vi "cam2 analyse.vi"() -> (0 "W6 chiffre":string, 1 "O6 chiffre":string, 2 "G1 chiffre":string, 3 "G4 chiffre":string, 4 "G8 chiffre":string, 5 "W9 chiffre":string, 7 "W8 chiffre":string, 9 "W7 chiffre":string, 11 "O3 chiffre":string, 12 "O9 chiffre":string, 13 "G2 chiffre":string, 14 "G7 chiffre":string)   [LabVIEW 2019]
uses:
  <vilib>/vision/Classification.llb/IMAQ Classifier Read Options.ctl
  <vilib>/vision/NI_Vision_Development_Module.lvlib
panel:
  in  "error in":errorcluster
  out "Coordinates":i32[](array[numeric])
  in  "G8":T1={"Global Rectangle"=[0, 0, 1279, 959], "Contours"=[{"ID"=enum."External", "Type"=3, "Coordinates"=[0, 0, 1279, 959]}]} {"Contours"."Type" items=["No Selection", "Point", "Line", "Rectangle", "Oval", "Polygon", "Freehand Region", "Annulus", "Unused2", "Unused3", "Broken Line", "Freehand Line", "Rotated Rectangle"]}
  out "G8":string[](array[string])
  in  "G7":T1={"Global Rectangle"=[0, 0, 1279, 959], "Contours"=[{"ID"=enum."External", "Type"=3, "Coordinates"=[0, 0, 1279, 959]}]} {"Contours"."Type" items=["No Selection", "Point", "Line", "Rectangle", "Oval", "Polygon", "Freehand Region", "Annulus", "Unused2", "Unused3", "Broken Line", "Freehand Line", "Rotated Rectangle"]}
  out "G7":string[](array[string])
  in  "G4":T1={"Global Rectangle"=[0, 0, 1279, 959], "Contours"=[{"ID"=enum."External", "Type"=3, "Coordinates"=[0, 0, 1279, 959]}]} {"Contours"."Type" items=["No Selection", "Point", "Line", "Rectangle", "Oval", "Polygon", "Freehand Region", "Annulus", "Unused2", "Unused3", "Broken Line", "Freehand Line", "Rotated Rectangle"]}
  out "G4":string[](array[string])
  in  "G2":T1={"Global Rectangle"=[0, 0, 1279, 959], "Contours"=[{"ID"=enum."External", "Type"=3, "Coordinates"=[0, 0, 1279, 959]}]} {"Contours"."Type" items=["No Selection", "Point", "Line", "Rectangle", "Oval", "Polygon", "Freehand Region", "Annulus", "Unused2", "Unused3", "Broken Line", "Freehand Line", "Rotated Rectangle"]}
  out "G2":string[](array[string])
  in  "G1":T1={"Global Rectangle"=[0, 0, 1279, 959], "Contours"=[{"ID"=enum."External", "Type"=3, "Coordinates"=[0, 0, 1279, 959]}]} {"Contours"."Type" items=["No Selection", "Point", "Line", "Rectangle", "Oval", "Polygon", "Freehand Region", "Annulus", "Unused2", "Unused3", "Broken Line", "Freehand Line", "Rotated Rectangle"]}
  out "G1":string[](array[string])
  in  "O9":T1={"Global Rectangle"=[0, 0, 1279, 959], "Contours"=[{"ID"=enum."External", "Type"=3, "Coordinates"=[0, 0, 1279, 959]}]} {"Contours"."Type" items=["No Selection", "Point", "Line", "Rectangle", "Oval", "Polygon", "Freehand Region", "Annulus", "Unused2", "Unused3", "Broken Line", "Freehand Line", "Rotated Rectangle"]}
  out "O9":string[](array[string])
  in  "O6":T1={"Global Rectangle"=[0, 0, 1279, 959], "Contours"=[{"ID"=enum."External", "Type"=3, "Coordinates"=[0, 0, 1279, 959]}]} {"Contours"."Type" items=["No Selection", "Point", "Line", "Rectangle", "Oval", "Polygon", "Freehand Region", "Annulus", "Unused2", "Unused3", "Broken Line", "Freehand Line", "Rotated Rectangle"]}
  out "O6":string[](array[string])
  in  "O3":T1={"Global Rectangle"=[0, 0, 1279, 959], "Contours"=[{"ID"=enum."External", "Type"=3, "Coordinates"=[0, 0, 1279, 959]}]} {"Contours"."Type" items=["No Selection", "Point", "Line", "Rectangle", "Oval", "Polygon", "Freehand Region", "Annulus", "Unused2", "Unused3", "Broken Line", "Freehand Line", "Rotated Rectangle"]}
  out "O3":string[](array[string])
  in  "W7":T1={"Global Rectangle"=[0, 0, 1279, 959], "Contours"=[{"ID"=enum."External", "Type"=3, "Coordinates"=[0, 0, 1279, 959]}]} {"Contours"."Type" items=["No Selection", "Point", "Line", "Rectangle", "Oval", "Polygon", "Freehand Region", "Annulus", "Unused2", "Unused3", "Broken Line", "Freehand Line", "Rotated Rectangle"]}
  out "W7":string[](array[string])
  in  "W8":T1={"Global Rectangle"=[0, 0, 1279, 959], "Contours"=[{"ID"=enum."External", "Type"=3, "Coordinates"=[0, 0, 1279, 959]}]} {"Contours"."Type" items=["No Selection", "Point", "Line", "Rectangle", "Oval", "Polygon", "Freehand Region", "Annulus", "Unused2", "Unused3", "Broken Line", "Freehand Line", "Rotated Rectangle"]}
  out "W8":string[](array[string])
  in  "W9":T1={"Global Rectangle"=[0, 0, 1279, 959], "Contours"=[{"ID"=enum."External", "Type"=3, "Coordinates"=[0, 0, 1279, 959]}]} {"Contours"."Type" items=["No Selection", "Point", "Line", "Rectangle", "Oval", "Polygon", "Freehand Region", "Annulus", "Unused2", "Unused3", "Broken Line", "Freehand Line", "Rotated Rectangle"]}
  out "W9":string[](array[string])
  in  "W6":T1={"Global Rectangle"=[640, 450, 686, 504], "Contours"=[{"ID"=enum."External", "Type"=3, "Coordinates"=[640, 450, 686, 504]}]} {"Contours"."Type" items=["No Selection", "Point", "Line", "Rectangle", "Oval", "Polygon", "Freehand Region", "Annulus", "Unused2", "Unused3", "Broken Line", "Freehand Line", "Rotated Rectangle"]}
  out "Image Out 2":T2(plugin-control)
  out "W6":string[](array[string])
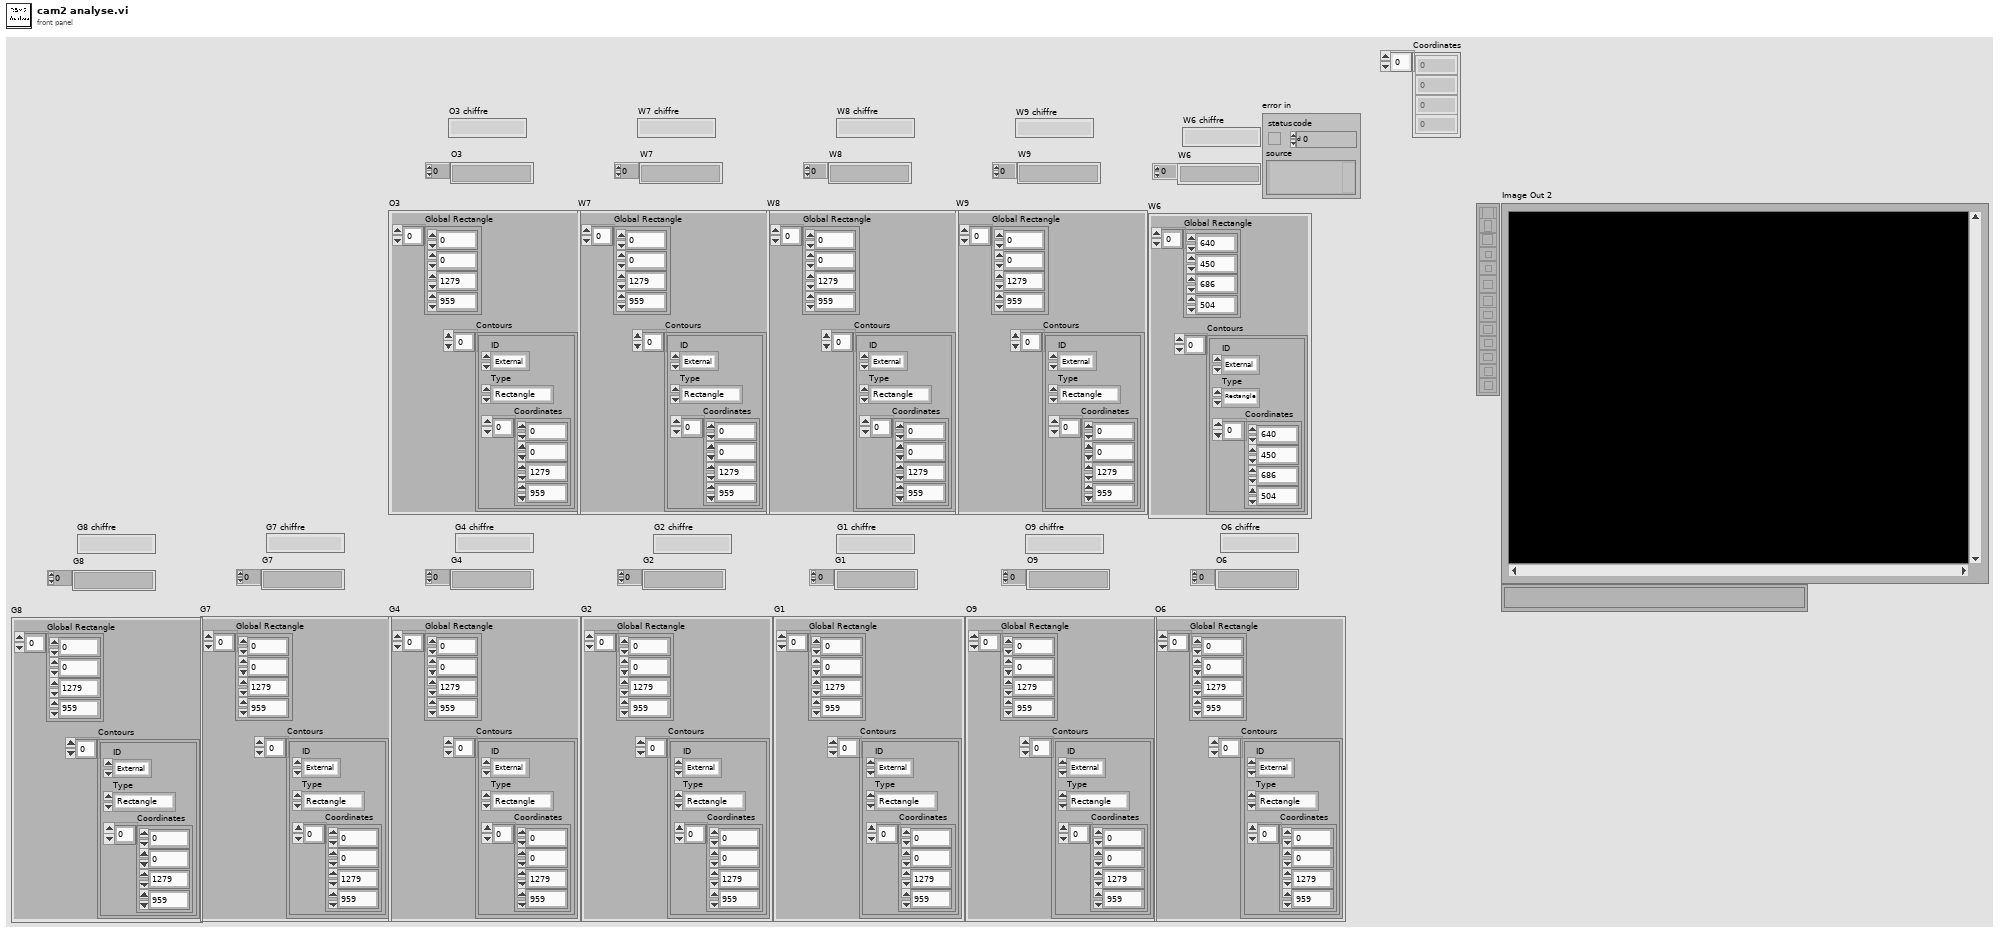
[diagram p1: front panel]
types:
  T1 = cluster{"Global Rectangle":i32[], "Contours":cluster{"ID":enum32{"External", "Internal"}, "Type":u32, "Coordinates":i32[]}[]}
  T2 = typedef "IMAQ Image.ctl" = refnum<image>
  T3 = typedef "IMAQ Classifier Read Options.ctl" = i32
  T4 = typedef "IMAQ Classifier Session.ctl" = refnum<k1>
  T5 = typedef "ROI Descriptor" = cluster{"Global Rectangle":i32[], "Contours":cluster{"ID":enum32{"External", "Internal"}, "Type":u32, "Coordinates":i32[]}[]}
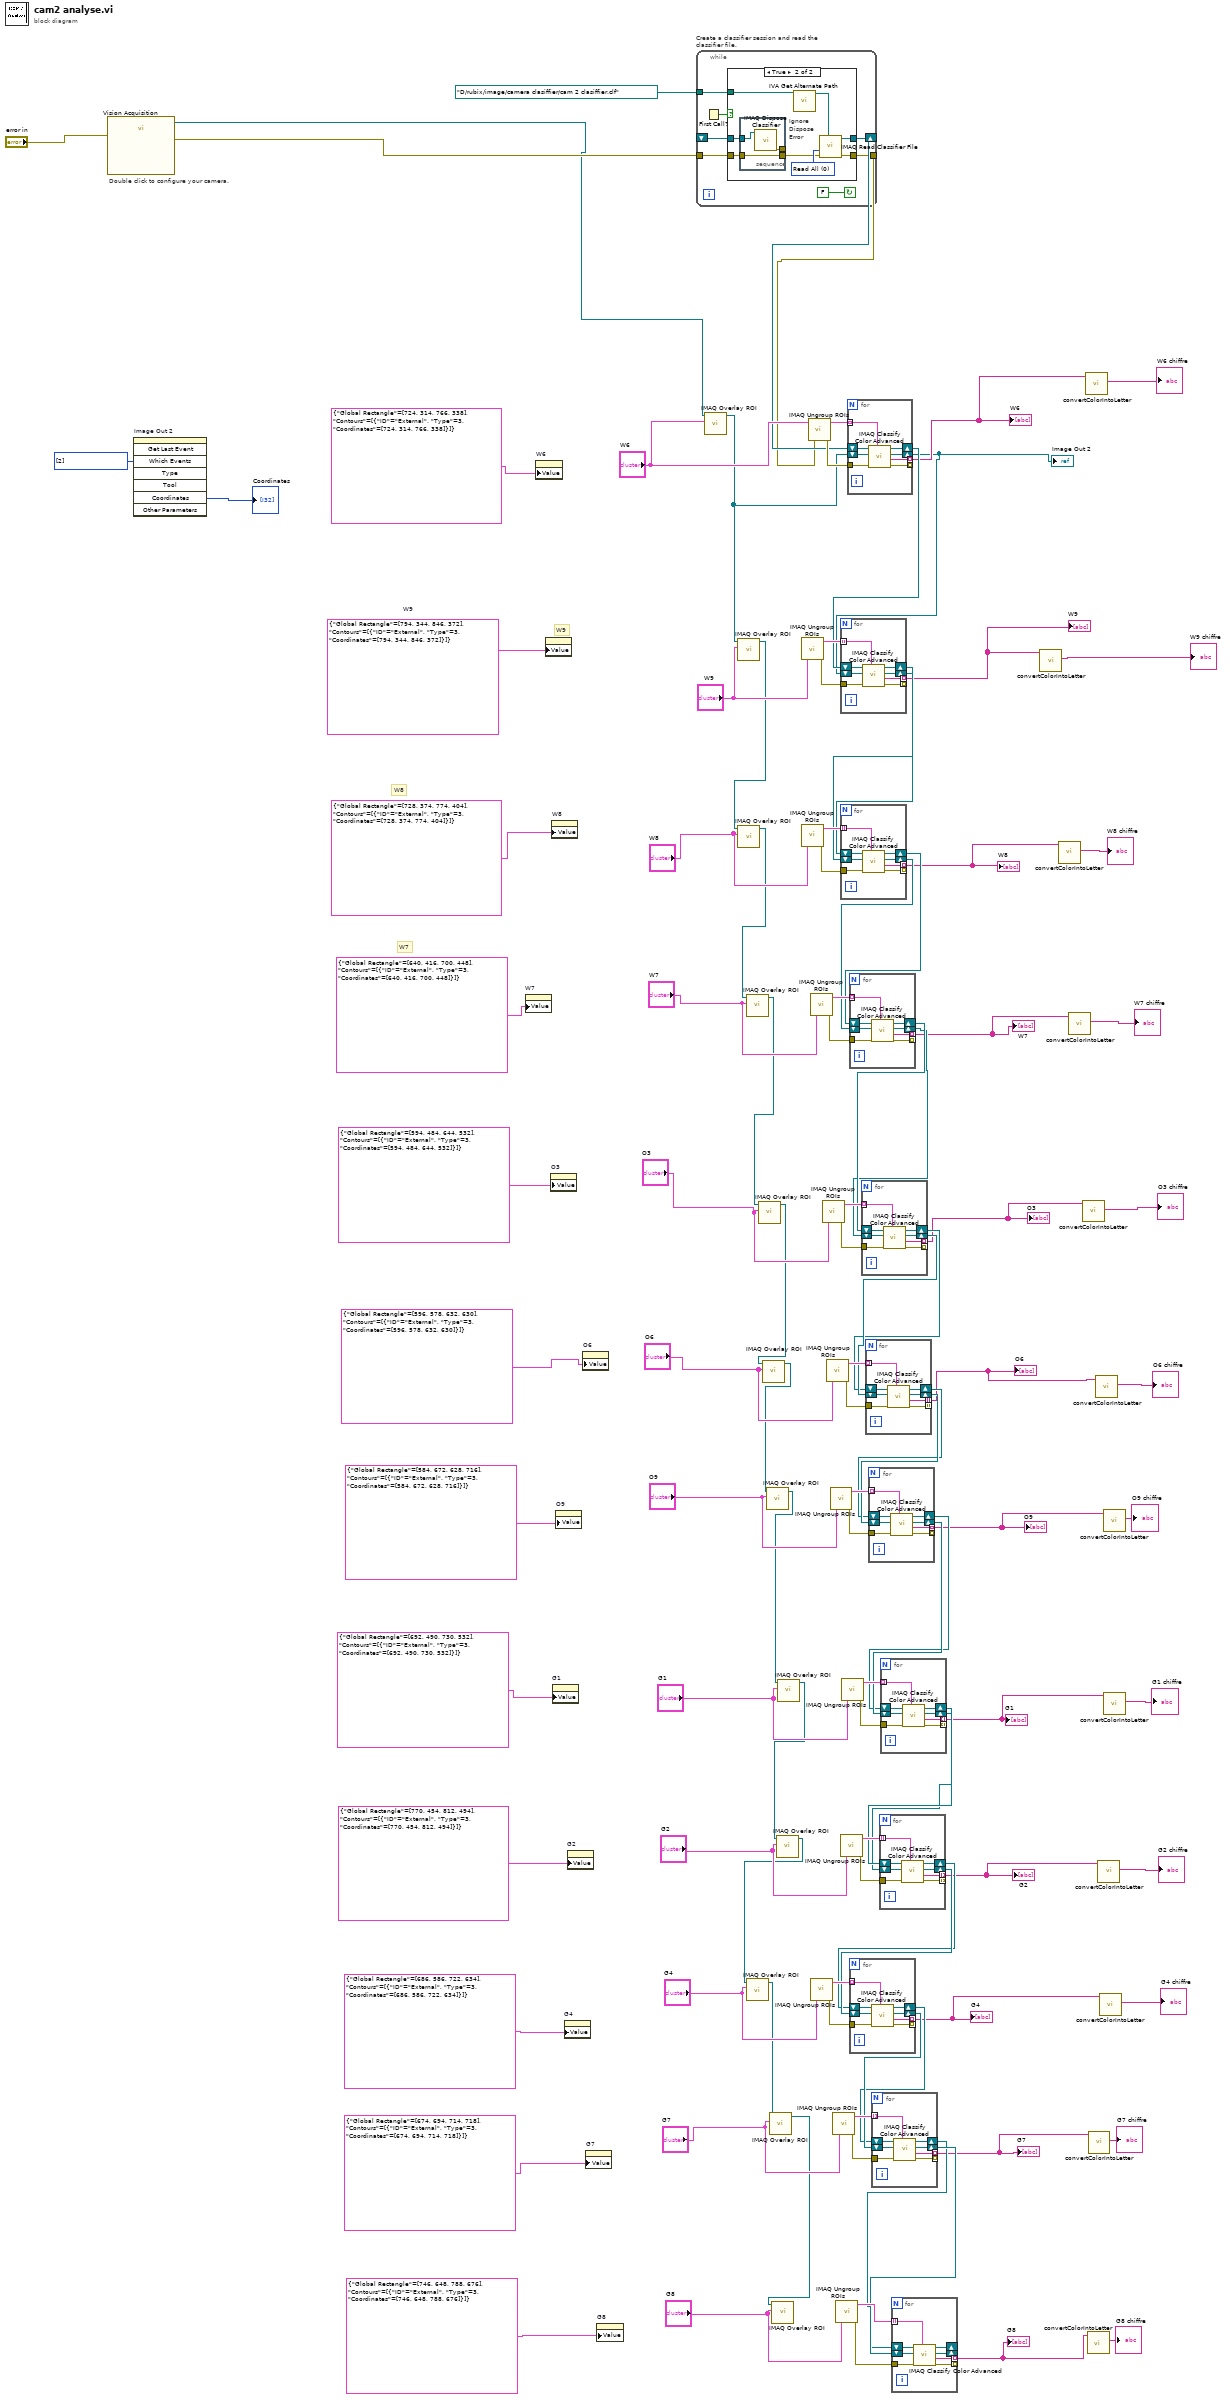
[diagram p0: block diagram]
diagram:
  w7 = i32[] [2] items=["No Event"=0, "Click Event"=1, "Draw Event"=2, "Size Event"=4, "Scroll Event"=5, "Double Click Event"=8] ("Which Events")
  # "W9"
  # "W7"
  # "W8"
  # "Double click to configure your camera."
  n1 = call "Vision Acquisition"("error in"="error in") -> ("Image Out"=w3:T2, "error out"=w113:errorcluster)  [unwired: 25 in]
  n2 = invoke on="Image Out 2" class="ImageControl" method="Get Last Event"("Which Events"=w7) -> ("Coordinates"=→"Coordinates":i32[])  [unwired: 7 in, 7 out]
  n3 = property on="W7" class="Clust (strict)"("Value"=T1 {"Global Rectangle"=[640, 416, 700, 448], "Contours"=[{"ID"=enum."External", "Type"=3, "Coordinates"=[640, 416, 700, 448]}]} ("ROI Descriptor (Color Classification 1)")) -> ()  [unwired: 2 in, 2 out]
  n4 = property on="W6" class="Clust (strict)"("Value"=T1 {"Global Rectangle"=[724, 314, 766, 338], "Contours"=[{"ID"=enum."External", "Type"=3, "Coordinates"=[724, 314, 766, 338]}]} ("ROI Descriptor (Color Classification 1)")) -> ()  [unwired: 2 in, 2 out]
  n5 = property on="W9" class="Clust (strict)"("Value"=T1 {"Global Rectangle"=[794, 344, 846, 372], "Contours"=[{"ID"=enum."External", "Type"=3, "Coordinates"=[794, 344, 846, 372]}]} ("ROI Descriptor (Color Classification 1)")) -> ()  [unwired: 2 in, 2 out]
  n6 = property on="O3" class="Clust (strict)"("Value"=T1 {"Global Rectangle"=[594, 484, 644, 532], "Contours"=[{"ID"=enum."External", "Type"=3, "Coordinates"=[594, 484, 644, 532]}]} ("ROI Descriptor (Color Classification 1)")) -> ()  [unwired: 2 in, 2 out]
  n7 = property on="W8" class="Clust (strict)"("Value"=T1 {"Global Rectangle"=[728, 374, 774, 404], "Contours"=[{"ID"=enum."External", "Type"=3, "Coordinates"=[728, 374, 774, 404]}]} ("ROI Descriptor (Color Classification 1)")) -> ()  [unwired: 2 in, 2 out]
  n8 = property on="G1" class="Clust (strict)"("Value"=T1 {"Global Rectangle"=[692, 490, 730, 532], "Contours"=[{"ID"=enum."External", "Type"=3, "Coordinates"=[692, 490, 730, 532]}]} ("ROI Descriptor (Color Classification 1)")) -> ()  [unwired: 2 in, 2 out]
  n9 = property on="O9" class="Clust (strict)"("Value"=T1 {"Global Rectangle"=[584, 672, 628, 716], "Contours"=[{"ID"=enum."External", "Type"=3, "Coordinates"=[584, 672, 628, 716]}]} ("ROI Descriptor (Color Classification 1)")) -> ()  [unwired: 2 in, 2 out]
  n10 = property on="G4" class="Clust (strict)"("Value"=T1 {"Global Rectangle"=[686, 586, 722, 634], "Contours"=[{"ID"=enum."External", "Type"=3, "Coordinates"=[686, 586, 722, 634]}]} ("ROI Descriptor (Color Classification 1)")) -> ()  [unwired: 2 in, 2 out]
  n11 = property on="G2" class="Clust (strict)"("Value"=T1 {"Global Rectangle"=[770, 454, 812, 494], "Contours"=[{"ID"=enum."External", "Type"=3, "Coordinates"=[770, 454, 812, 494]}]} ("ROI Descriptor (Color Classification 1)")) -> ()  [unwired: 2 in, 2 out]
  n12 = property on="O6" class="Clust (strict)"("Value"=T1 {"Global Rectangle"=[596, 578, 632, 630], "Contours"=[{"ID"=enum."External", "Type"=3, "Coordinates"=[596, 578, 632, 630]}]} ("ROI Descriptor (Color Classification 1)")) -> ()  [unwired: 2 in, 2 out]
  n13 = property on="G7" class="Clust (strict)"("Value"=T1 {"Global Rectangle"=[674, 694, 714, 718], "Contours"=[{"ID"=enum."External", "Type"=3, "Coordinates"=[674, 694, 714, 718]}]} ("ROI Descriptor (Color Classification 1)")) -> ()  [unwired: 2 in, 2 out]
  n14 = property on="G8" class="Clust (strict)"("Value"=T1 {"Global Rectangle"=[746, 648, 788, 676], "Contours"=[{"ID"=enum."External", "Type"=3, "Coordinates"=[746, 648, 788, 676]}]} ("ROI Descriptor (Color Classification 1)")) -> ()  [unwired: 2 in, 2 out]
  n15 = while "Create a classifier session and read the classifier file." {
    shift-right: [w120] -> w6
    shift-left: _ -> [w119]
    tunnel: w113 -> [w117]
    tunnel: [w116] -> w5
    tunnel: path "D:/rubix/image/camera clasiffier/cam 2 clasiffier.clf" ("File Path") -> [w115]
    stop <- FALSE continue-if-true
    n16 = First Call?() -> (First Call?: T/F=w114:bool)
    n17 = case shown="True" w114 {
      tunnel: [w122 w129] -> w120
      tunnel: w119 -> [w122 w127]
      tunnel: w117 -> [w121 w126]
      tunnel: [w121 w128] -> w116
      tunnel: w115 -> [_ w124]
      frame False {
      }
      frame True {
        w130 = T3 0 items=["Read All", "Add Samples, Do Not Change Options", "Read Options, Do Not Add Samples"] ("Read Options")
        # "Ignore Dispose Error"
        n18 = stacked-sequence {
          tunnel: w127 -> [w133]
          tunnel: w126 -> [w132]
          tunnel: [w132] -> w125
          tunnel: [w131] -> _
          frame #0 {
            n19 = call "IMAQ Dispose Classifier"("Classifier Session"=w133) -> ("error out"=w131:errorcluster)  [unwired: 1 in, 9 out]
          }
        }
        n20 = call <vilib>:"IVA Get Alternate Path.vi"("Path In"=w124) -> ("Path Out"=w123:path)  [unwired: 10 out]
        n21 = call "IMAQ Read Classifier File"("File Path"=w123, "error in (no error)"=w125, "Read Options"=w130) -> ("error out"=w128:errorcluster, "Classifier Session"=w129:T4)  [unwired: 1 in, 6 out]
      }
    }
  }
  n22 = call "IMAQ Overlay ROI"("ROI Descriptor"="W6", "Image"=w3) -> ("Image Out"=w4:T2)  [unwired: 8 in, 1 out]
  n23 = call "IMAQ Overlay ROI"("ROI Descriptor"="W9", "Image"=w4) -> ("Image Out"=w103:T2)  [unwired: 8 in, 1 out]
  n24 = call "IMAQ Overlay ROI"("ROI Descriptor"="W8", "Image"=w103) -> ("Image Out"=w95:T2)  [unwired: 8 in, 1 out]
  n25 = call "IMAQ Overlay ROI"("ROI Descriptor"="W7", "Image"=w95) -> ("Image Out"=w87:T2)  [unwired: 8 in, 1 out]
  n26 = call "IMAQ Overlay ROI"("ROI Descriptor"="O3", "Image"=w87) -> ("Image Out"=w80:T2)  [unwired: 8 in, 1 out]
  n27 = call "IMAQ Overlay ROI"("ROI Descriptor"="O6", "Image"=w80) -> ("Image Out"=w75:T2)  [unwired: 8 in, 1 out]
  n28 = call "IMAQ Overlay ROI"("ROI Descriptor"="O9", "Image"=w75) -> ("Image Out"=w68:T2)  [unwired: 8 in, 1 out]
  n29 = call "IMAQ Overlay ROI"("ROI Descriptor"="G1", "Image"=w68) -> ("Image Out"=w58:T2)  [unwired: 8 in, 1 out]
  n30 = call "IMAQ Overlay ROI"("ROI Descriptor"="G2", "Image"=w58) -> ("Image Out"=w54:T2)  [unwired: 8 in, 1 out]
  n31 = call "IMAQ Overlay ROI"("ROI Descriptor"="G4", "Image"=w54) -> ("Image Out"=w45:T2)  [unwired: 8 in, 1 out]
  n32 = call "IMAQ Overlay ROI"("ROI Descriptor"="G7", "Image"=w45) -> ("Image Out"=w40:T2)  [unwired: 8 in, 1 out]
  n33 = call "IMAQ Overlay ROI"("ROI Descriptor"="G8", "Image"=w40) -> ()  [unwired: 8 in, 2 out]
  n34 = call "IMAQ Ungroup ROIs"("ROI Descriptor"="W9") -> ("error out"=w109:errorcluster, "ROI Descriptors out"=w108:T5[])  [unwired: 1 in, 2 out]
  n35 = call "IMAQ Ungroup ROIs"("ROI Descriptor"="W8") -> ("error out"=w105:errorcluster, "ROI Descriptors out"=w104:T5[])  [unwired: 1 in, 2 out]
  n36 = call "IMAQ Ungroup ROIs"("error in (no error)"=w5, "ROI Descriptor"="W6") -> ("error out"=w111:errorcluster, "ROI Descriptors out"=w110:T5[])  [unwired: 2 out]
  n37 = call "IMAQ Ungroup ROIs"("ROI Descriptor"="W7") -> ("error out"=w98:errorcluster, "ROI Descriptors out"=w97:T5[])  [unwired: 1 in, 2 out]
  n38 = call "IMAQ Ungroup ROIs"("ROI Descriptor"="G4") -> ("error out"=w57:errorcluster, "ROI Descriptors out"=w56:T5[])  [unwired: 1 in, 2 out]
  n39 = call "IMAQ Ungroup ROIs"("ROI Descriptor"="O3") -> ("error out"=w91:errorcluster, "ROI Descriptors out"=w90:T5[])  [unwired: 1 in, 2 out]
  n40 = call "IMAQ Ungroup ROIs"("ROI Descriptor"="O6") -> ("error out"=w84:errorcluster, "ROI Descriptors out"=w83:T5[])  [unwired: 1 in, 2 out]
  n41 = call "IMAQ Ungroup ROIs"("ROI Descriptor"="O9") -> ("error out"=w78:errorcluster, "ROI Descriptors out"=w77:T5[])  [unwired: 1 in, 2 out]
  n42 = call "IMAQ Ungroup ROIs"("ROI Descriptor"="G7") -> ("error out"=w50:errorcluster, "ROI Descriptors out"=w49:T5[])  [unwired: 1 in, 2 out]
  n43 = call "IMAQ Ungroup ROIs"("ROI Descriptor"="G8") -> ("error out"=w43:errorcluster, "ROI Descriptors out"=w42:T5[])  [unwired: 1 in, 2 out]
  n44 = call "IMAQ Ungroup ROIs"("ROI Descriptor"="G2") -> ("error out"=w64:errorcluster, "ROI Descriptors out"=w63:T5[])  [unwired: 1 in, 2 out]
  n45 = call "IMAQ Ungroup ROIs"("ROI Descriptor"="G1") -> ("error out"=w71:errorcluster, "ROI Descriptors out"=w70:T5[])  [unwired: 1 in, 2 out]
  n46 = for {
    tunnel: [w141] -> w13 mode=indexing
    tunnel: [w140] -> _ mode=indexing
    tunnel: w111 -> [w138]
    tunnel: w110 -> [w137] mode=indexing
    shift-right: [w135] -> w2
    shift-left: w4 -> [w136]
    shift-right: [w134] -> w15
    shift-left: w6 -> [w139]
    n47 = call "IMAQ Classify Color Advanced"("ROI Descriptor"=w137, "error in (no error)"=w138, "Image"=w136, "Classifier Session"=w139) -> ("error out"=w140:errorcluster, "Class"=w141:string, "Image (dup)"=w135:T2, "Classifier Session (dup)"=w134:T4)  [unwired: 4 out]
  }
  "W6" <- w13
  "Image Out 2" <- w2
  n48 = for {
    tunnel: [w149] -> w10 mode=indexing
    tunnel: [w148] -> _ mode=indexing
    tunnel: w109 -> [w146]
    tunnel: w108 -> [w145] mode=indexing
    shift-right: [w143] -> w101
    shift-left: w2 -> [w144]
    shift-right: [w142] -> w102
    shift-left: w15 -> [w147]
    n49 = call "IMAQ Classify Color Advanced"("ROI Descriptor"=w145, "error in (no error)"=w146, "Image"=w144, "Classifier Session"=w147) -> ("error out"=w148:errorcluster, "Class"=w149:string, "Image (dup)"=w143:T2, "Classifier Session (dup)"=w142:T4)  [unwired: 4 out]
  }
  "W9" <- w10
  n50 = for {
    tunnel: [w157] -> w35 mode=indexing
    tunnel: [w156] -> _ mode=indexing
    tunnel: w105 -> [w154]
    tunnel: w104 -> [w153] mode=indexing
    shift-right: [w151] -> w94
    shift-left: w101 -> [w152]
    shift-right: [w150] -> w93
    shift-left: w102 -> [w155]
    n51 = call "IMAQ Classify Color Advanced"("ROI Descriptor"=w153, "error in (no error)"=w154, "Image"=w152, "Classifier Session"=w155) -> ("error out"=w156:errorcluster, "Class"=w157:string, "Image (dup)"=w151:T2, "Classifier Session (dup)"=w150:T4)  [unwired: 4 out]
  }
  "W8" <- w35
  n52 = for {
    tunnel: [w165] -> w34 mode=indexing
    tunnel: [w164] -> _ mode=indexing
    tunnel: w98 -> [w162]
    tunnel: w97 -> [w161] mode=indexing
    shift-right: [w159] -> w88
    shift-left: w94 -> [w160]
    shift-right: [w158] -> w89
    shift-left: w93 -> [w163]
    n53 = call "IMAQ Classify Color Advanced"("ROI Descriptor"=w161, "error in (no error)"=w162, "Image"=w160, "Classifier Session"=w163) -> ("error out"=w164:errorcluster, "Class"=w165:string, "Image (dup)"=w159:T2, "Classifier Session (dup)"=w158:T4)  [unwired: 4 out]
  }
  "W7" <- w34
  n54 = for {
    tunnel: [w173] -> w33 mode=indexing
    tunnel: [w172] -> _ mode=indexing
    tunnel: w91 -> [w170]
    tunnel: w90 -> [w169] mode=indexing
    shift-right: [w167] -> w82
    shift-left: w88 -> [w168]
    shift-right: [w166] -> w81
    shift-left: w89 -> [w171]
    n55 = call "IMAQ Classify Color Advanced"("ROI Descriptor"=w169, "error in (no error)"=w170, "Image"=w168, "Classifier Session"=w171) -> ("error out"=w172:errorcluster, "Class"=w173:string, "Image (dup)"=w167:T2, "Classifier Session (dup)"=w166:T4)  [unwired: 4 out]
  }
  "O3" <- w33
  n56 = for {
    tunnel: [w181] -> w32 mode=indexing
    tunnel: [w180] -> _ mode=indexing
    tunnel: w84 -> [w178]
    tunnel: w83 -> [w177] mode=indexing
    shift-right: [w175] -> w74
    shift-left: w82 -> [w176]
    shift-right: [w174] -> w73
    shift-left: w81 -> [w179]
    n57 = call "IMAQ Classify Color Advanced"("ROI Descriptor"=w177, "error in (no error)"=w178, "Image"=w176, "Classifier Session"=w179) -> ("error out"=w180:errorcluster, "Class"=w181:string, "Image (dup)"=w175:T2, "Classifier Session (dup)"=w174:T4)  [unwired: 4 out]
  }
  "O6" <- w32
  n58 = for {
    tunnel: [w189] -> w31 mode=indexing
    tunnel: [w188] -> _ mode=indexing
    tunnel: w78 -> [w186]
    tunnel: w77 -> [w185] mode=indexing
    shift-right: [w183] -> w67
    shift-left: w74 -> [w184]
    shift-right: [w182] -> w66
    shift-left: w73 -> [w187]
    n59 = call "IMAQ Classify Color Advanced"("ROI Descriptor"=w185, "error in (no error)"=w186, "Image"=w184, "Classifier Session"=w187) -> ("error out"=w188:errorcluster, "Class"=w189:string, "Image (dup)"=w183:T2, "Classifier Session (dup)"=w182:T4)  [unwired: 4 out]
  }
  "O9" <- w31
  n60 = for {
    tunnel: [w197] -> w30 mode=indexing
    tunnel: [w196] -> _ mode=indexing
    tunnel: w71 -> [w194]
    tunnel: w70 -> [w193] mode=indexing
    shift-right: [w191] -> w61
    shift-left: w67 -> [w192]
    shift-right: [w190] -> w62
    shift-left: w66 -> [w195]
    n61 = call "IMAQ Classify Color Advanced"("ROI Descriptor"=w193, "error in (no error)"=w194, "Image"=w192, "Classifier Session"=w195) -> ("error out"=w196:errorcluster, "Class"=w197:string, "Image (dup)"=w191:T2, "Classifier Session (dup)"=w190:T4)  [unwired: 4 out]
  }
  "G1" <- w30
  n62 = for {
    tunnel: [w205] -> w29 mode=indexing
    tunnel: [w204] -> _ mode=indexing
    tunnel: w64 -> [w202]
    tunnel: w63 -> [w201] mode=indexing
    shift-right: [w199] -> w53
    shift-left: w61 -> [w200]
    shift-right: [w198] -> w52
    shift-left: w62 -> [w203]
    n63 = call "IMAQ Classify Color Advanced"("ROI Descriptor"=w201, "error in (no error)"=w202, "Image"=w200, "Classifier Session"=w203) -> ("error out"=w204:errorcluster, "Class"=w205:string, "Image (dup)"=w199:T2, "Classifier Session (dup)"=w198:T4)  [unwired: 4 out]
  }
  "G2" <- w29
  n64 = for {
    tunnel: [w213] -> w28 mode=indexing
    tunnel: [w212] -> _ mode=indexing
    tunnel: w57 -> [w210]
    tunnel: w56 -> [w209] mode=indexing
    shift-right: [w207] -> w48
    shift-left: w53 -> [w208]
    shift-right: [w206] -> w47
    shift-left: w52 -> [w211]
    n65 = call "IMAQ Classify Color Advanced"("ROI Descriptor"=w209, "error in (no error)"=w210, "Image"=w208, "Classifier Session"=w211) -> ("error out"=w212:errorcluster, "Class"=w213:string, "Image (dup)"=w207:T2, "Classifier Session (dup)"=w206:T4)  [unwired: 4 out]
  }
  "G4" <- w28
  n66 = for {
    tunnel: [w221] -> w27 mode=indexing
    tunnel: [w220] -> _ mode=indexing
    tunnel: w50 -> [w218]
    tunnel: w49 -> [w217] mode=indexing
    shift-right: [w215] -> w39
    shift-left: w48 -> [w216]
    shift-right: [w214] -> w38
    shift-left: w47 -> [w219]
    n67 = call "IMAQ Classify Color Advanced"("ROI Descriptor"=w217, "error in (no error)"=w218, "Image"=w216, "Classifier Session"=w219) -> ("error out"=w220:errorcluster, "Class"=w221:string, "Image (dup)"=w215:T2, "Classifier Session (dup)"=w214:T4)  [unwired: 4 out]
  }
  "G7" <- w27
  n68 = for {
    tunnel: [w229] -> w26 mode=indexing
    tunnel: [w228] -> _ mode=indexing
    tunnel: w43 -> [w226]
    tunnel: w42 -> [w225] mode=indexing
    shift-right: [w223] -> _
    shift-left: w39 -> [w224]
    shift-right: [w222] -> _
    shift-left: w38 -> [w227]
    n69 = call "IMAQ Classify Color Advanced"("ROI Descriptor"=w225, "error in (no error)"=w226, "Image"=w224, "Classifier Session"=w227) -> ("error out"=w228:errorcluster, "Class"=w229:string, "Image (dup)"=w223:T2, "Classifier Session (dup)"=w222:T4)  [unwired: 4 out]
  }
  "G8" <- w26
  n70 = call "convertColorIntoLetter.vi"("Array"=w10) -> ("String"=→"W9 chiffre":string)  [unwired: 10 in]
  n71 = call "convertColorIntoLetter.vi"("Array"=w35) -> ("String"=→"W8 chiffre":string)  [unwired: 10 in]
  n72 = call "convertColorIntoLetter.vi"("Array"=w34) -> ("String"=→"W7 chiffre":string)  [unwired: 10 in]
  n73 = call "convertColorIntoLetter.vi"("Array"=w33) -> ("String"=→"O3 chiffre":string)  [unwired: 10 in]
  n74 = call "convertColorIntoLetter.vi"("Array"=w13) -> ("String"=→"W6 chiffre":string)  [unwired: 10 in]
  n75 = call "convertColorIntoLetter.vi"("Array"=w26) -> ("String"=→"G8 chiffre":string)  [unwired: 10 in]
  n76 = call "convertColorIntoLetter.vi"("Array"=w27) -> ("String"=→"G7 chiffre":string)  [unwired: 10 in]
  n77 = call "convertColorIntoLetter.vi"("Array"=w32) -> ("String"=→"O6 chiffre":string)  [unwired: 10 in]
  n78 = call "convertColorIntoLetter.vi"("Array"=w29) -> ("String"=→"G2 chiffre":string)  [unwired: 10 in]
  n79 = call "convertColorIntoLetter.vi"("Array"=w28) -> ("String"=→"G4 chiffre":string)  [unwired: 10 in]
  n80 = call "convertColorIntoLetter.vi"("Array"=w31) -> ("String"=→"O9 chiffre":string)  [unwired: 10 in]
  n81 = call "convertColorIntoLetter.vi"("Array"=w30) -> ("String"=→"G1 chiffre":string)  [unwired: 10 in]
